vi "AH Bridge Wait Times.vi"(11 "Frequency":dbl=1000.0) -> (1 "Frequency Out":dbl, 2 "Averaging Time":string[](array[string]), 3 "Wait Time (mS)":u32[](array[numeric]))   [LabVIEW 2024]
uses:
  <vilib>/gmath/NI_Gmath.lvlib
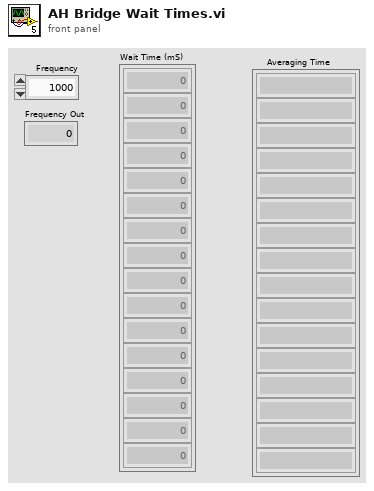
[diagram p1: front panel]
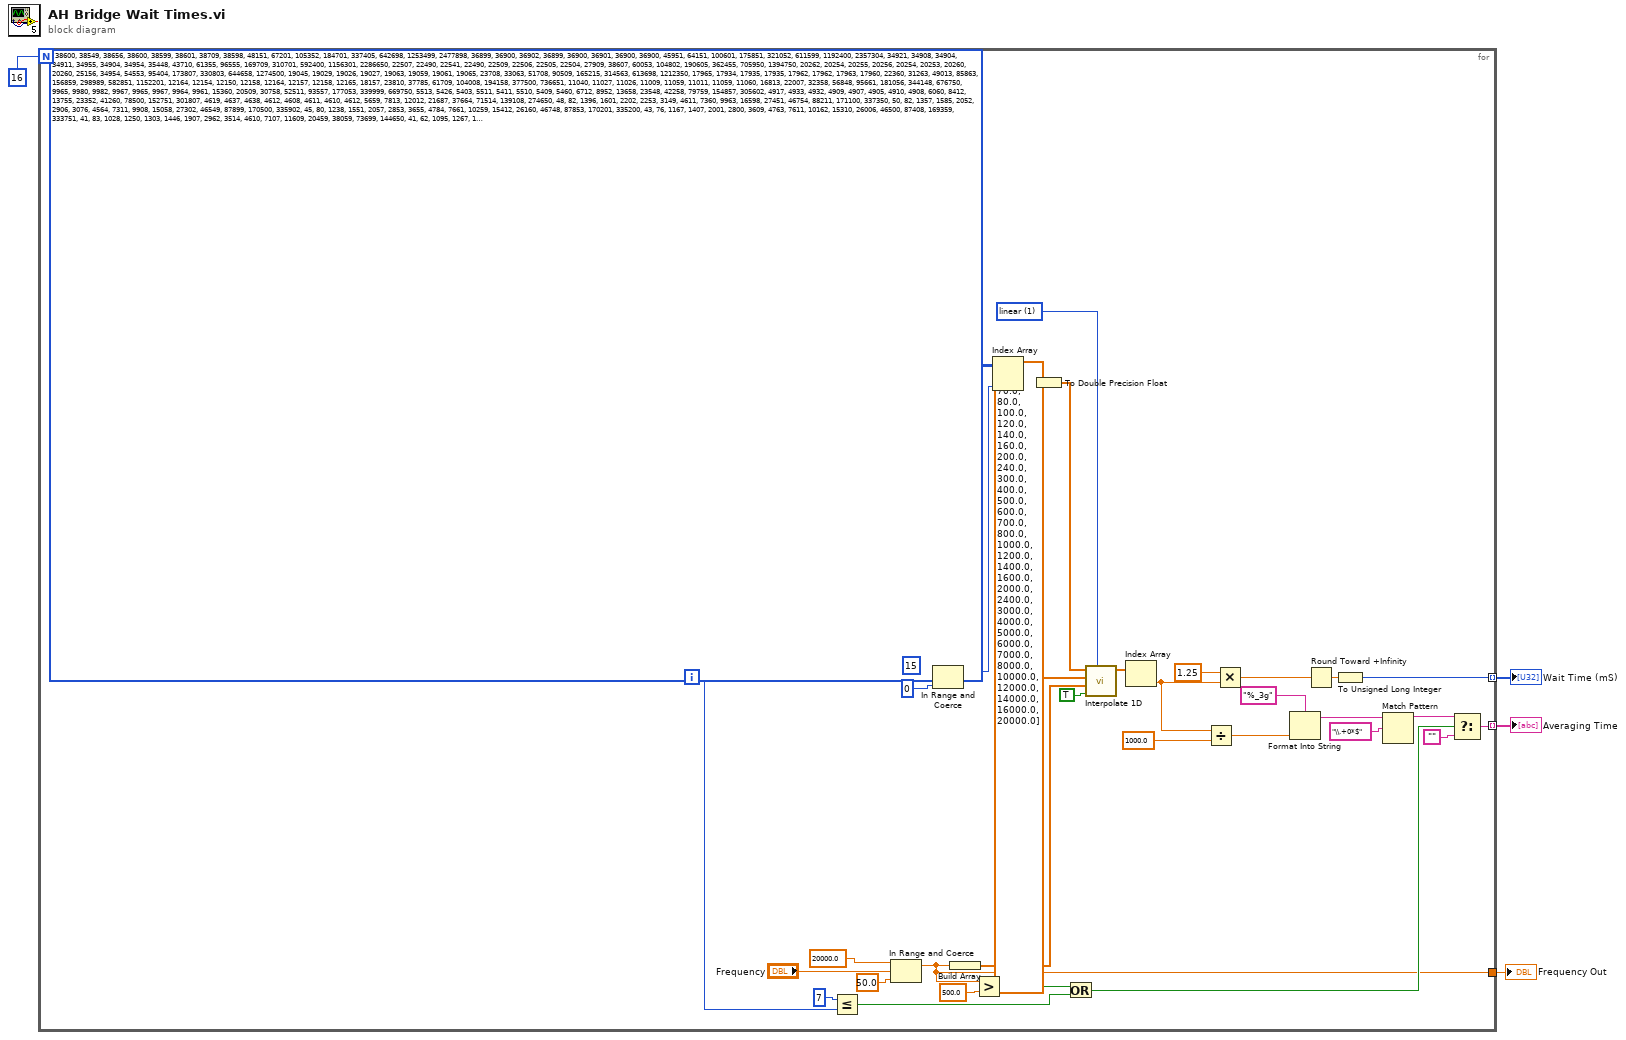
[diagram p0: block diagram]
diagram:
  n1 = for {
    N: 16 -> [_]
    tunnel: [w29] -> w4 mode=indexing
    tunnel: [w10] -> w2 mode=indexing
    tunnel: [w7] -> w1
    i -> [w14]
    w34 = 1 items=["nearest", "linear", "spline", "cubic Hermite", "Lagrange"] ("method")
    n2 = Less Or Equal?(x=7, y=w14) -> (x <= y?=w18:bool)
    n3 = In Range and Coerce(upper limit=20000.0, x="Frequency", lower limit=50.0) -> (coerced(x)=w7:dbl)  [unwired: 1 out]
    n4 = In Range and Coerce(upper limit=15 ("lower limit"), x=w14, lower limit=0 ("upper limit")) -> (coerced(x)=w28:i32)  [unwired: 1 out]
    n5 = Build Array(w7) -> (w37:dbl[])
    n6 = Greater?(x=w7, y=500.0) -> (0:w12:bool)
    n7 = Index Array(array=u32[][] [[38600, 38549, 38656, 38600, 38599, 38601, 38709, 38598, 48151, 67201, 105352, 184701, 337405, 642698, 1253499, 2477898], [36899, 36900, 36902, 36899, 36900, 36901, 36900, 36900, 45951, 64151, 100601, 175851, 321052, 611599, 1192400, 2357304], [34921, 34908, 34904, 34911, 34955, 34904, 34954, 35448, 43710, 61355, 96555, 169709, 310701, 592400, 1156301, 2286650], [22507, 22490, 22541, 22490, 22509, 22506, 22505, 22504, 27909, 38607, 60053, 104802, 190605, 362455, 705950, 1394750], [20262, 20254, 20255, 20256, 20254, 20253, 20260, 20260, 25156, 34954, 54553, 95404, 173807, 330803, 644658, 1274500], [19045, 19029, 19026, 19027, 19063, 19059, 19061, 19065, 23708, 33063, 51708, 90509, 165215, 314563, 613698, 1212350], [17965, 17934, 17935, 17935, 17962, 17962, 17963, 17960, 22360, 31263, 49013, 85863, 156859, 298989, 582851, 1152201], [12164, 12154, 12150, 12158, 12164, 12157, 12158, 12165, 18157, 23810, 37785, 61709, 104008, 194158, 377500, 736651], [11040, 11027, 11026, 11009, 11059, 11011, 11059, 11060, 16813, 22007, 32358, 56848, 95661, 181056, 344148, 676750], [9965, 9980, 9982, 9967, 9965, 9967, 9964, 9961, 15360, 20509, 30758, 52511, 93557, 177053, 339999, 669750], [5513, 5426, 5403, 5511, 5411, 5510, 5409, 5460, 6712, 8952, 13658, 23548, 42258, 79759, 154857, 305602], [4917, 4933, 4932, 4909, 4907, 4905, 4910, 4908, 6060, 8412, 13755, 23352, 41260, 78500, 152751, 301807], [4619, 4637, 4638, 4612, 4608, 4611, 4610, 4612, 5659, 7813, 12012, 21687, 37664, 71514, 139108, 274650], [48, 82, 1396, 1601, 2202, 2253, 3149, 4611, 7360, 9963, 16598, 27451, 46754, 88211, 171100, 337350], [50, 82, 1357, 1585, 2052, 2906, 3076, 4564, 7311, 9908, 15058, 27302, 46549, 87899, 170500, 335902], [45, 80, 1238, 1551, 2057, 2853, 3655, 4784, 7661, 10259, 15412, 26160, 46748, 87853, 170201, 335200], [43, 76, 1167, 1407, 2001, 2800, 3609, 4763, 7611, 10162, 15310, 26006, 46500, 87408, 169359, 333751], [41, 83, 1028, 1250, 1303, 1446, 1907, 2962, 3514, 4610, 7107, 11609, 20459, 38059, 73699, 144650], [41, 62, 1095, 1267, 1390, 1599, 1970, 3153, 3758, 4859, 7058, 11561, 20354, 37905, 73000, 143349], [58, 79, 1019, 1176, 1224, 1655, 1881, 3058, 3563, 4610, 6517, 10557, 18563, 34511, 66307, 130202], [56, 59, 980, 1116, 1158, 1557, 1837, 3012, 3509, 4460, 6511, 10559, 18510, 34408, 66265, 129900], [56, 59, 934, 1072, 1104, 1254, 1861, 2650, 3460, 4497, 6460, 10562, 18414, 34363, 65951, 130150], [38, 58, 924, 1107, 1104, 1259, 1910, 2697, 3407, 4412, 6407, 10461, 18409, 34361, 66262, 130099], [38, 55, 919, 968, 1238, 1539, 1754, 2663, 3462, 4362, 6400, 10557, 18451, 37750, 66009, 129750], [37, 51, 1128, 979, 1276, 1376, 1250, 1924, 2614, 3110, 4061, 6106, 10061, 17859, 33557, 64961], [38, 1306, 1306, 1120, 1038, 1113, 1519, 1909, 2549, 3158, 4063, 6111, 10009, 17858, 33511, 64860], [36, 1307, 1306, 1132, 987, 1540, 1931, 1881, 2612, 3061, 4058, 6113, 9914, 17748, 33460, 64813], [37, 1306, 1305, 1250, 1316, 1588, 2110, 1882, 2612, 3063, 4060, 6113, 9962, 17807, 33457, 64756], [37, 1306, 1305, 986, 1257, 1319, 1470, 1772, 2561, 3011, 3958, 6007, 9913, 17749, 33409, 64700], [37, 50, 1305, 926, 1284, 1250, 2172, 1810, 2511, 3012, 4005, 6011, 9957, 17754, 33352, 64658], [47, 1306, 1125, 978, 1259, 1235, 1810, 1802, 2558, 3001, 4161, 6050, 9907, 17701, 33301, 64607], [37, 1306, 1093, 1250, 1306, 1337, 2037, 1922, 2561, 3116, 4010, 6099, 9960, 17706, 33362, 64450], [37, 50, 1306, 1260, 1170, 1346, 1855, 1923, 2609, 3114, 4059, 6057, 9959, 17710, 33208, 64356]] ("AH2700A Wait Times"), index (col)=w28) -> (element=w32:u32[])  [unwired: 1 in]
    n8 = To Double Precision Float(number=w32) -> (double precision float=w23:dbl[])
    n9 = Or(x=w12, y=w18) -> (x .or. y?=w16:bool)
    n10 = call <vilib>:"Interpolate 1D.vi"("method"=w34, "X is monotonic"=TRUE, "xi"=w37, "X"=dbl[] [50.0, 60.0, 70.0, 80.0, 100.0, 120.0, 140.0, 160.0, 200.0, 240.0, 300.0, 400.0, 500.0, 600.0, 700.0, 800.0, 1000.0, 1200.0, 1400.0, 1600.0, 2000.0, 2400.0, 3000.0, 4000.0, 5000.0, 6000.0, 7000.0, 8000.0, 10000.0, 12000.0, 14000.0, 16000.0, 20000.0], "Y"=w23) -> ("yi"=w31:dbl[])  [unwired: 4 in, 2 out]
    n11 = Index Array(array=w31) -> (element=w11:dbl)  [unwired: 1 in]
    n12 = Divide(x=w11, y=1000.0) -> (x/y=w9:dbl)
    n13 = Multiply(x=1.25, y=w11) -> (x*y=w6:dbl)
    n14 = Format Into String(format string="%_3g", w9) -> (resulting string=w21:string)  [unwired: 2 in, 1 out]
    n15 = Round Toward +Infinity(x=w6) -> (ceil(x): smallest int >= x=w30:dbl)
    n16 = To Unsigned Long Integer(number=w30) -> (unsigned 32bit integer=w29:u32)
    n17 = Match Pattern(string=w21, regular expression="\\.+0*$") -> (before substring=w17:string)  [unwired: 1 in, 3 out]
    n18 = Select(t=w17, s=w16, f="") -> (s? t:f=w10:string)
  }
  "Wait Time (mS)" <- w4
  "Averaging Time" <- w2
  "Frequency Out" <- w1
